vi "get_centering.vi"(0 "ScanModeTS090821Circular2D in":refnum<class "ImagingModeTS090821Circular2D.lvclass">, 5 "error in (no error)":errorcluster) -> (14 "ScanModeTS090821Circular2D out":refnum<class "ImagingModeTS090821Circular2D.lvclass">, 15 "x center":dbl, 16 "y center":dbl, 18 "rotation angle":dbl, 19 "error out":errorcluster)   [LabVIEW 2010, in "ImagingModeTS090821Circular2D.lvclass"]
uses:
  ImagingModeTS090821Circular2D.lvclass
  ImagingModeTS090821Circular2D.lvclass/ImagingModeTS090821Circular2D.ctl
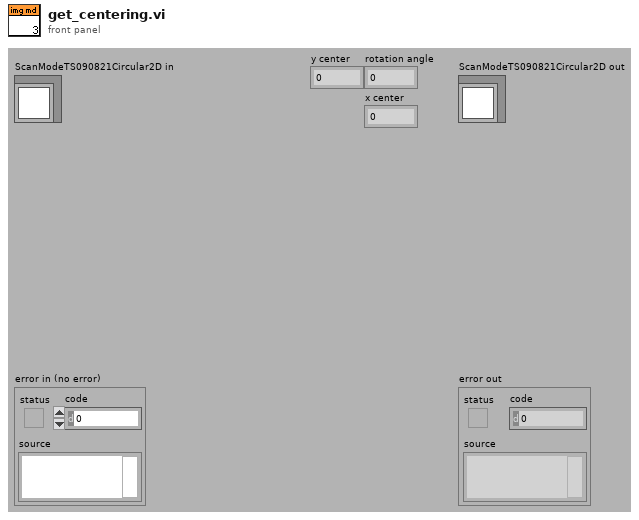
[diagram p1: front panel]
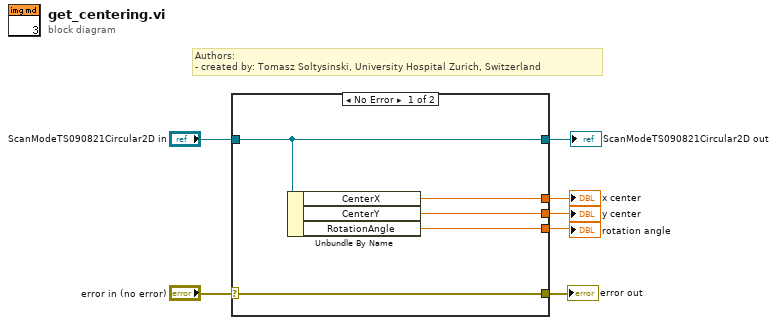
[diagram p0: block diagram]
diagram:
  # "Authors: \n- created by: Tomasz Soltysinski, University Hospital Zurich, Switzerland"
  n1 = case shown="No Error" "error in (no error)" {
    selector: "error in (no error)" -> [w12 w14]
    tunnel: [w12 w14] -> w6
    tunnel: [w11 w13] -> w4
    tunnel: "ScanModeTS090821Circular2D in" -> [w11 w13]
    tunnel: [w10 _] -> w3
    tunnel: [w9 _] -> w2
    tunnel: [w8 _] -> w1
    frame No Error {
      n2 = Unbundle By Name(w11) -> ("CenterX"=w10:dbl, "CenterY"=w9:dbl, "RotationAngle"=w8:dbl)
    }
    frame Error {
    }
  }
  "error out" <- w6
  "ScanModeTS090821Circular2D out" <- w4
  "x center" <- w3
  "y center" <- w2
  "rotation angle" <- w1
